vi "4x7Display.vi"(7 "Display Length":i32, 8 "Error In":errorcluster, 9 "Input":u32=4, 10 "Custom Command Number":u16=6, 11 "LINX Resource In":T1) -> (0 "Error Out":errorcluster, 3 "LINX Resource Out":T1)   [LabVIEW 2022 SP3]
doc: "Custom Command 7 is for the Score Display. Custom Command 8 is for the Time Display. Custom Command 9 is for Combo Display. Sends number to display to the applicable 7 segment display."
uses:
  <vilib>/MakerHub/LINX/Private/Type Defs/LINX Ref.ctl
  <vilib>/MakerHub/LINX/Private/Type Defs/Platform.ctl
  <vilib>/MakerHub/LINX/Private/Type Defs/Interface.ctl
  <vilib>/MakerHub/LINX/Private/Device/Type Defs/LINX Device Config.ctl
  <vilib>/MakerHub/LINX/Private/Device/Type Defs/TCP Config.ctl
  <vilib>/MakerHub/LINX/Private/Device/Type Defs/Channels.ctl
  <vilib>/MakerHub/LINX/LMH-LINX.lvlib
  <vilib>/MakerHub/LINX/Private/Device/Device.lvlib
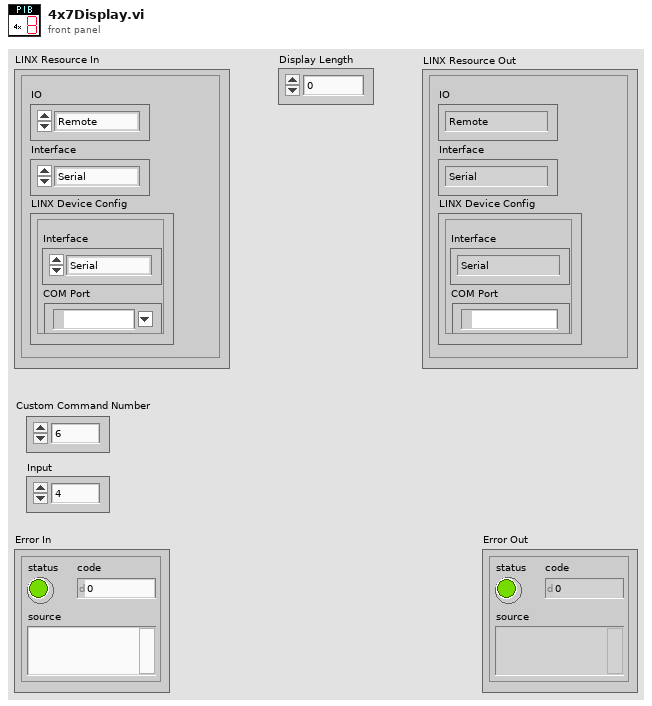
[diagram p1: front panel]
types:
  T1 = typedef "LMH-LINX.lvlib/LINX Ref.ctl" = cluster{"IO":T2, "Interface":T3, "LINX Device Config":T4}
  T2 = typedef "LMH-LINX.lvlib/Platform.ctl" = enum16{"Remote", "Local"}
  T3 = typedef "LMH-LINX.lvlib/Interface.ctl" = enum16{"Serial", "TCP"}
  T4 = typedef "LMH-LINX.lvlib/Device.lvlib/LINX Device Config.ctl" = cluster{"Interface":T3, "COM Port":refnum<visa-resource-name>, "TCP Configuration":T5, "Device Family":u8, "Device ID":u8, "Device Name":string, "TCP Ref":refnum<k5>, "Channels":T6}
  T5 = typedef "LMH-LINX.lvlib/Device.lvlib/TCP Config.ctl" = cluster{"IP Address":string, "Port":u16}
  T6 = typedef "LMH-LINX.lvlib/Channels.ctl" = cluster{"DI":u8[], "DO":u8[], "AI":u8[], "AO":u8[], "PWM":u8[], "QE":u8[], "UART":u8[], "I2C 2":u8[], "SPI":u8[], "CAN":u8[], "Servo":u8[], "AI Ref (V)":dbl, "AI Resolution (Bits)":u8, "AO Ref (V)":dbl, "AO Resolution (Bits)":u8}
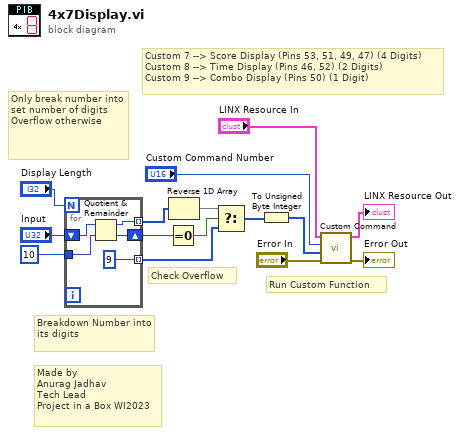
[diagram p0: block diagram]
diagram:
  # "Made by \nAnurag Jadhav\nTech Lead\nProject in a Box WI2023"
  # "Custom 7 --> Score Display (Pins 53, 51, 49, 47) (4 Digits)\nCustom 8 --> Time Display (Pins 46, 52) (2 Digits)\nCustom 9 --> Combo Display (Pins 50) (1 Digit)"
  # "Run Custom Function"
  # "Check Overflow"
  # "Only break number into set number of digits\nOverflow otherwise"
  # "Breakdown Number into its digits"
  n1 = for {
    N: "Display Length" -> [_]
    tunnel: u32 10 -> [w16]
    tunnel: [w18] -> w10 mode=indexing
    tunnel: [u32 9] -> w11 mode=indexing
    shift-right: [w19] -> w9
    shift-left: "Input" -> [w20]
    n2 = Quotient & Remainder(x=w20, y=w16) -> (x-y*floor(x/y)=w18:u32, floor(x/y)=w19:u32)
  }
  n3 = Equal To 0?(x=w9) -> (x = 0?=w12:bool)
  n4 = Reverse 1D Array(array=w10) -> (reversed array=w13:u32[])
  n5 = Select(t=w13, s=w12, f=w11) -> (s? t:f=w14:u32[])
  n6 = To Unsigned Byte Integer(number=w14) -> (unsigned 8bit integer=w7:u8[])
  n7 = call <vilib>:"Custom Command.vi"("Error In"="Error In", "Data"=w7, "Custom Command Number"="Custom Command Number", "LINX Resource"="LINX Resource In") -> ("Error Out"=→"Error Out":errorcluster, "LINX Resource"=→"LINX Resource Out":T1)  [unwired: 4 in, 2 out]
